vi "Actor Core.vi"(8 "error in":errorcluster, 11 "Integrate in":refnum<class "Integrate.lvclass">) -> (0 "error out":errorcluster, 3 "Actor out":refnum<class "Actor.lvclass">)   [LabVIEW 2015, in "Integrate.lvclass"]
doc: "(<B>Filename</B>: Actor Framework.lvlib:Actor.lvclass:Actor Core.vi)\n\nReceives messages to the actor, reacts to them, and initiates any error handling that may shut the actor down.\n\nDescendant classes may override this VI to append parallel tasks for the actor to complete while it handles messages. Overrides use the Call Parent Method node."
uses:
  Integrate.lvclass
  <vilib>/ActorFramework/Actor/Actor.lvclass
  Integrator Configuration.ctl
  NHMFL_Core/Libraries/Utilities/Controls/Integrate channel.ctl
  Measure_core/Process Object/Process Object.lvclass
panel:
  in  "Configuration":T1={"Integrate"=[{"Channel"="Bdot", "Output name"="Field", "Factor"=1.0, "Start time"=nan, "Duration"=nan}], "Offset duration "=0.0095, "TDMS group name"="p"} {"Integrate"."Duration" format="%#_6p"; "Integrate"."Start time" format="%#_6p"}
  # "Input CH            Factor      Output CH      Start         Duration"
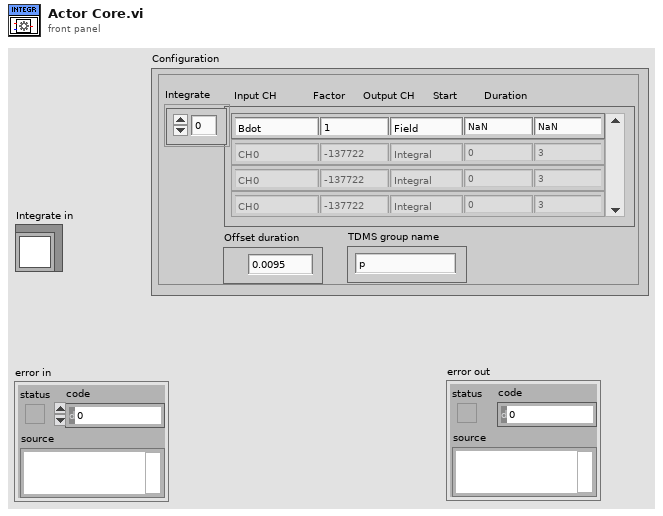
[diagram p1: front panel]
types:
  T1 = typedef "Integrator Configuration.ctl" = cluster{"Integrate":T2[], "Offset duration ":dbl, "TDMS group name":string}
  T2 = typedef "Integrate channel.ctl" = cluster{"Channel":string, "Output name":string, "Factor":dbl, "Start time":dbl, "Duration":dbl}
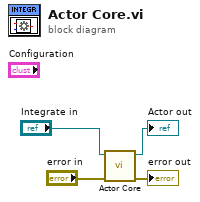
[diagram p0: block diagram]
diagram:
  n1 = call-parent "Actor Core.vi"("error in"="error in", "Measure Object in"="Integrate in") -> ("error out"=→"error out":errorcluster, "Actor out"=→"Actor out":refnum<class "Actor.lvclass">)  [unwired: 8 in]
